vi "input.vi"(8 "error in (no error)":errorcluster, 9 "Frequncey [Hz]":u16=1 min=1 max=10 step=1, 10 "Duty Cycle [%]":dbl=50.0 min=0.0 max=100.0 format="%#_13g", 11 "controller in":refnum<class "controller.lvclass">) -> (0 "error out":errorcluster, 3 "controller out":refnum<class "controller.lvclass">)   [LabVIEW 2025, in "controller.lvclass"]
uses:
  controller.lvclass
  controller.lvclass/controller.ctl
  <vilib>/DAQmx/write.llb/DAQmx Write (Digital Bool 1Line 1Point).vi
  <vilib>/DAQmx/miscellaneous.llb/DAQmx Fill In Error Info.vi
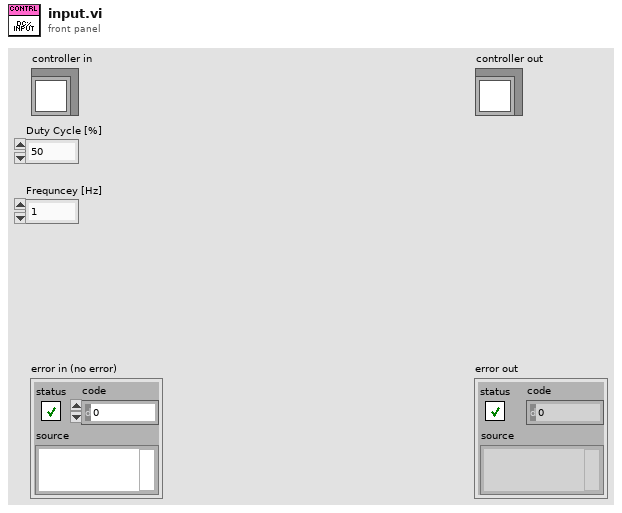
[diagram p1: front panel]
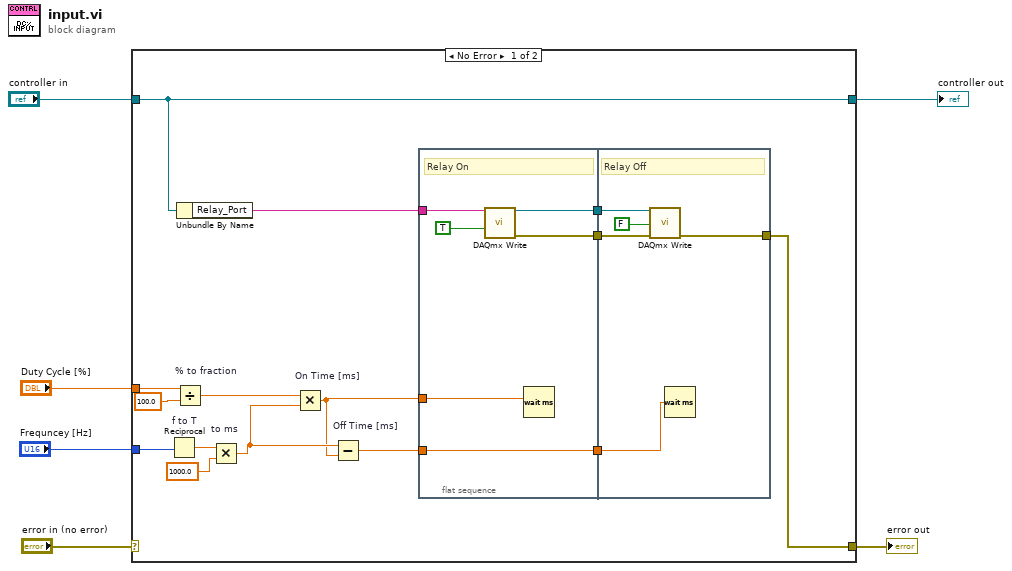
[diagram p0: block diagram]
diagram:
  n1 = case shown="No Error" "error in (no error)" {
    selector: "error in (no error)" -> [_ w34]
    tunnel: [w7 w34] -> w5
    tunnel: [w11 w33] -> w3
    tunnel: "controller in" -> [w11 w33]
    tunnel: "Duty Cycle [%]" -> [w20 _]
    tunnel: "Frequncey [Hz]" -> [w21 _]
    frame No Error {
      n2 = Reciprocal "f to T"(x=w21) -> (1/x=w17:dbl)
      n3 = Divide "% to fraction"(x=w20, y=100.0) -> (x/y=w18:dbl)
      n4 = Unbundle By Name(w11) -> ("Relay_Port"=w10:string)
      n5 = Multiply "to ms"(x=w17, y=1000.0 ("value")) -> (x*y=w15:dbl)
      n6 = Multiply "On Time [ms]"(x=w18, y=w15) -> (x*y=w14:dbl)
      n7 = Subtract "Off Time [ms]"(x=w15, y=w14) -> (x-y=w12:dbl)
      n8 = flat-sequence {
        tunnel: w14 -> [w27]
        tunnel: [w26] -> w13
        tunnel: w12 -> [w26]
        tunnel: w10 -> [w25]
        tunnel: [w23] -> w9
        tunnel: [w22] -> w8
        tunnel: w13 -> [w32]
        tunnel: w9 -> [w31]
        tunnel: w8 -> [w30]
        tunnel: [w28] -> w7
        frame #0 {
          # "Relay On"
          n9 = call-poly <vilib>:"DAQmx Write.vi"("task/channels in"=w25, "data"=TRUE) -> ("task out"=w23:refnum<k21>, "error out"=w22:errorcluster)  [unwired: 11 in, 1 out]
          n10 = Wait (ms)(milliseconds to wait=w27) -> ()  [unwired: 1 out]
        }
        frame #1 {
          # "Relay Off"
          n11 = call-poly <vilib>:"DAQmx Write.vi"("task/channels in"=w31, "data"=FALSE, "error in"=w30) -> ("error out"=w28:errorcluster)  [unwired: 10 in, 2 out]
          n12 = Wait (ms)(milliseconds to wait=w32) -> ()  [unwired: 1 out]
        }
      }
    }
    frame Error {
    }
  }
  "error out" <- w5
  "controller out" <- w3
